vi "GetDigitalType.vi"(8 "error in (no error)":errorcluster, 11 "Control in":refnum<vi>) -> (0 "error out":errorcluster, 2 "String":string, 3 "Control in 2":refnum<vi>)   [LabVIEW 2014]
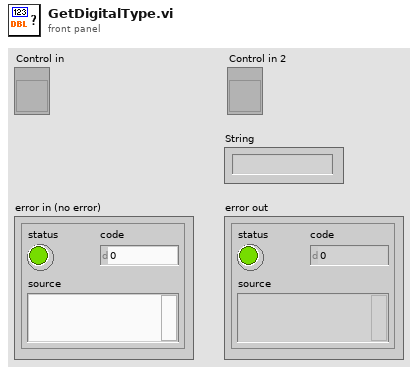
[diagram p1: front panel]
types:
  T1 = typedef "LVNumericRepresentation.ctl" = enum32{"Extended Precision", "Double Precision", "Single Precision", "Long", "Word", "Byte", "Unsigned Long", "Unsigned Word", "Unsigned Byte", "Complex Extended", "Complex Double", "Complex Single", "Quad", "Unsigned Quad", "Fixed-Point"}
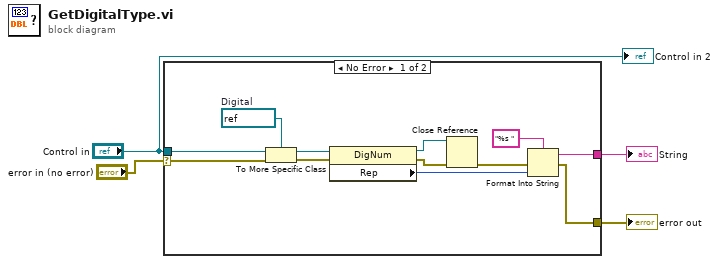
[diagram p0: block diagram]
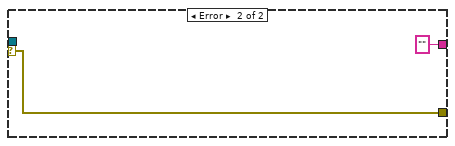
[diagram p2: hidden frame]
diagram:
  n1 = case shown="No Error" "error in (no error)" {
    selector: "error in (no error)" -> [w5 w18]
    tunnel: [w16 w18] -> w4
    tunnel: "Control in" -> [w14 _]
    tunnel: [w13 ""] -> w2
    frame No Error {
      w10 = refnum<vi> refnum  # Digital
      n2 = To More Specific Class(target class=w10, reference=w14, error in=w5) -> (specific class reference=w8:refnum<vi>, error out=w9:errorcluster)
      n3 = property class="DigNum"(reference=w8, error in=w9) -> (reference out=w6:refnum<vi>, error out=w15:errorcluster, "Rep"=w12:T1)
      n4 = Close Reference(reference=w6, error in (no error)=w15) -> (error out=w7:errorcluster)
      n5 = Format Into String(format string="%s ", error in=w7, w12) -> (resulting string=w13:string, error out=w16:errorcluster)  [unwired: 1 in]
    }
    frame Error {
    }
  }
  "error out" <- w4
  "String" <- w2
  "Control in 2" <- "Control in"
